vi "Save scan settings.vi"(8 "Path":path, 10 "New scan settings":T1={"Light intensity (Suns)"=1.0, "Pre-bias time (s)"=0.0, "Maximum voltage (V)"=0.0, "Minimum voltage (V)"=1.4, "Range Options"=0, "1st scan FB to SC?"=TRUE, "Step Size (V)"=0.0, "Source Delay (s)"=0.0, "Inverted device"=FALSE, "Measure stabilized power output"=FALSE, "Stabilzation time (s)"=0.0, "Use Vmp from JV scan"=FALSE, "Stabization voltage (V)"=0.0, "Only stabilize best pixels"=TRUE, "Number of pixels to stabilize \nper substrate"=0, "Stabilization time step (s)"=1.0, "Use max power tracking"=FALSE, "Pre-bias voltage (V)"=-1.4, "No. of data point averages"=1.0, "No. of J-V averages"=1.0, "Integration time (ms)"=200.0} {"Number of pixels to stabilize \nper substrate" items=["1", "2", "3", "4", "5", "6", "7", "8"]; "Range Options" items=["Auto Range", "Semi-Auto Range", "100 uA", "1 mA", "10 mA", "100 mA", "1A"]}, 11 "New name":string) -> ()   [LabVIEW 2011]
uses:
  Typedefs/Scan settings.ctl
  <vilib>/Utility/file.llb/Write To Spreadsheet File (string).vi
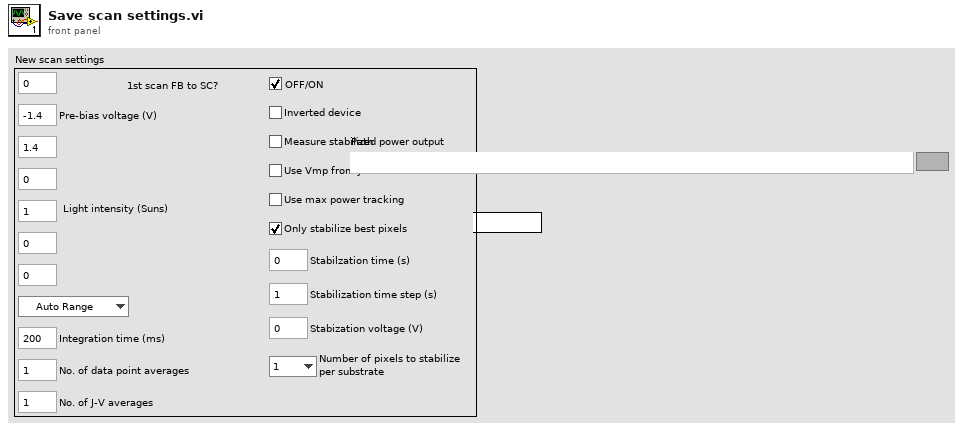
[diagram p1: front panel]
types:
  T1 = typedef "Scan settings.ctl" = cluster{"Light intensity (Suns)":dbl, "Pre-bias time (s)":dbl, "Maximum voltage (V)":dbl, "Minimum voltage (V)":dbl, "Range Options":u16, "1st scan FB to SC?":bool, "Step Size (V)":dbl, "Source Delay (s)":dbl, "Inverted device":bool, "Measure stabilized power output":bool, "Stabilzation time (s)":dbl, "Use Vmp from JV scan":bool, "Stabization voltage (V)":dbl, "Only stabilize best pixels":bool, "Number of pixels to stabilize \nper substrate":u16, "Stabilization time step (s)":dbl, "Use max power tracking":bool, "Pre-bias voltage (V)":dbl, "No. of data point averages":dbl, "No. of J-V averages":dbl, "Integration time (ms)":dbl}
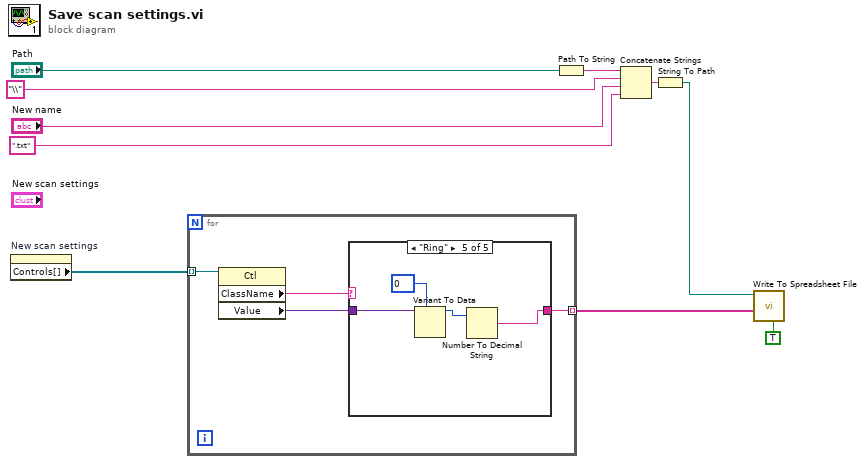
[diagram p0: block diagram]
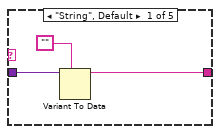
[diagram p2: hidden frame]
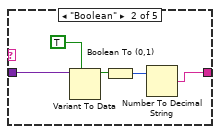
[diagram p3: hidden frame]
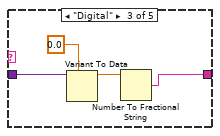
[diagram p4: hidden frame]
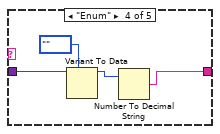
[diagram p5: hidden frame]
diagram:
  n1 = property on="New scan settings" class="Clust (strict)"() -> ("Controls[]"=w4:refnum<vi>[])  [unwired: 2 in, 2 out]
  n2 = for {
    tunnel: w4 -> [w14] mode=indexing
    tunnel: [w11] -> w2 mode=indexing
    n3 = property class="Ctl"(reference=w14) -> ("ClassName"=w13:string, "Value"=w12:variant)  [unwired: 1 in, 2 out]
    n4 = case shown="\"Ring\"" w13 {
      tunnel: w12 -> [w17 w22 w26 w30 w32]
      tunnel: [w15 w18 w23 w27 w31] -> w11
      frame "String", Default {
        n5 = Variant To Data(type="", Variant=w17) -> (data=w15:string)  [unwired: 1 in, 1 out]
      }
      frame "Boolean" {
        n6 = Variant To Data(type=TRUE, Variant=w22) -> (data=w20:bool)  [unwired: 1 in, 1 out]
        n7 = Boolean To (0,1)(Boolean=w20) -> (0, 1=w19:i16)
        n8 = Number To Decimal String(number=w19) -> (decimal integer string=w18:string)  [unwired: 1 in]
      }
      frame "Digital" {
        n9 = Variant To Data(type=0.0, Variant=w26) -> (data=w24:dbl)  [unwired: 1 in, 1 out]
        n10 = Number To Fractional String(number=w24) -> (F-format string=w23:string)  [unwired: 3 in]
      }
      frame "Enum" {
        n11 = Variant To Data(type=enum16{""}."", Variant=w30) -> (data=w28:enum16{""})  [unwired: 1 in, 1 out]
        n12 = Number To Decimal String(number=w28) -> (decimal integer string=w27:string)  [unwired: 1 in]
      }
      frame "Ring" {
        w34 = u16 0 items=[""]
        n13 = Variant To Data(type=w34, Variant=w32) -> (data=w33:u16)  [unwired: 1 in, 1 out]
        n14 = Number To Decimal String(number=w33) -> (decimal integer string=w31:string)  [unwired: 1 in]
      }
    }
  }
  n15 = Path To String(path="Path") -> (string=w10:string)
  n16 = Concatenate Strings(w10, "\\", "New name", ".txt" ("y")) -> (w9:string)
  n17 = String To Path(string=w9) -> (path=w3:path)
  n18 = call-poly <vilib>:"Write To Spreadsheet File.vi"("transpose? (no:F)"=TRUE, "1D data"=w2, "file path (dialog if empty)"=w3) -> ()  [unwired: 5 in, 1 out]
